vi "Get TDC Count.vi"(8 "error in (no error)":errorcluster, 11 "TDCManager":T1) -> (0 "error out":errorcluster, 2 "Count":i32, 3 "TDCManager out":T1)   [LabVIEW 2016, in "HPTDC Driver Library.lvlib"]
uses:
  HPTDC Driver Library.lvlib
  Typedefs/TDCManager.ctl
  C:/Users/CRT Controller/CRTC Labview Application/Source/HPTDC Driver Library Folder/Library files/hptdc_net4_3.7.0_x64.dll
  hptdc_net4_3.7.0_x64.dll
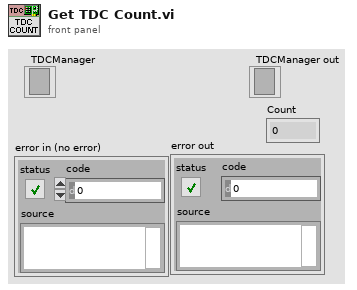
[diagram p1: front panel]
types:
  T1 = typedef "HPTDC Driver Library.lvlib/TDCManager.ctl" = refnum<k24>
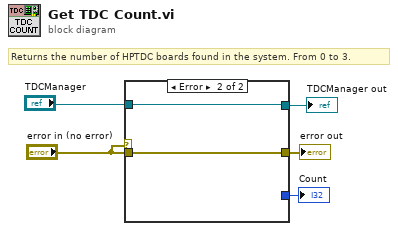
[diagram p0: block diagram]
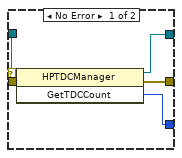
[diagram p2: hidden frame]
diagram:
  # "Returns the number of HPTDC boards found in the system. From 0 to 3."
  n1 = case shown="Error" "error in (no error)" {
    tunnel: "error in (no error)" -> [w10 w11]
    tunnel: [w9 w11] -> w5
    tunnel: [w8 _] -> w4
    tunnel: "TDCManager" -> [w7 w12]
    tunnel: [w6 w12] -> w2
    frame No Error {
      n2 = invoke class="HPTDCManager" method="GetTDCCount"(reference=w7, error in=w10) -> (reference out=w6:T1, error out=w9:errorcluster, "GetTDCCount"=w8:i32)  [unwired: 1 in]
    }
    frame Error {
    }
  }
  "error out" <- w5
  "Count" <- w4
  "TDCManager out" <- w2
